vi "AMZ_S3_AUTH_Add or Replace Authorization Header.vi"(8 "error in (no error)":errorcluster, 10 "Authorization Header value":string, 11 "Headers in":T1[](array[typedef])) -> (0 "error out":errorcluster, 3 "Headers":T1[](array[typedef]))   [LabVIEW 2015, in "LV Interface for Amazon S3.lvlib"]
uses:
  LV Interface for Amazon S3.lvlib
  Typedefs/AMZ_S3_HTTP Header-Value pair.ctl
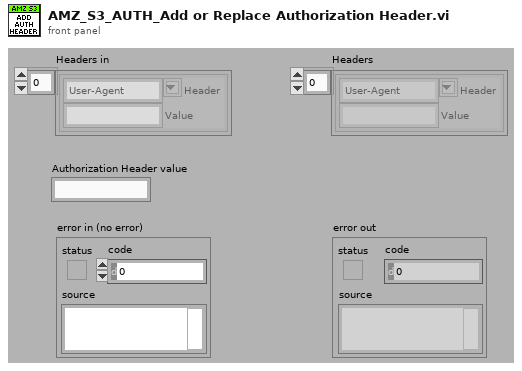
[diagram p1: front panel]
types:
  T1 = typedef "LV Interface for Amazon S3.lvlib/AMZ_S3_HTTP Header-Value pair.ctl" = cluster{"Header":string, "Value":string}
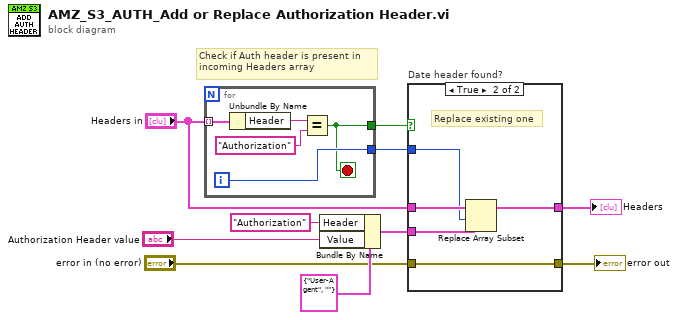
[diagram p0: block diagram]
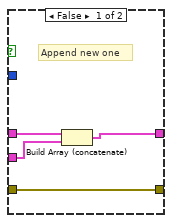
[diagram p2: hidden frame]
diagram:
  # "Check if Auth header is present in\nincoming Headers array"
  n1 = for {
    tunnel: "Headers in" -> [w15] mode=indexing
    tunnel: [w12] -> w8
    tunnel: [w11] -> w10
    i -> [w12]
    stop <- w11 stop-if-true
    n2 = Unbundle By Name(w15) -> ("Header"=w14:string)
    n3 = Equal?(x=w14, y="Authorization") -> (x = y?=w11:bool)
  }
  n4 = Bundle By Name(cluster=T1 {"Header"="User-Agent", "Value"=""} ("HTTP Header-Value pair"), "Header"="Authorization", "Value"="Authorization Header value") -> (w5:T1)
  n5 = case "Date header found?" shown="True" w10 {
    tunnel: "Headers in" -> [w19 w24]
    tunnel: w8 -> [_ w23]
    tunnel: [w17 w22] -> w4
    tunnel: "error in (no error)" -> [w16 w20]
    tunnel: w5 -> [w18 w21]
    tunnel: [w16 w20] -> w3
    frame False {
      # "Append new one"
      n6 = Build Array (concatenate)(w19, w18) -> (w17:T1[])
    }
    frame True {
      # "Replace existing one"
      n7 = Replace Array Subset(array=w24, new element=w21, index=w23) -> (w22:T1[])
    }
  }
  "Headers" <- w4
  "error out" <- w3
